vi "Write Tree Control Ref.vi"(8 "error in (no error)":errorcluster, 10 "Tag Tree Reference":refnum<vi>, 11 "Tag Tree Helper In":refnum<class "Tag Tree Helper.lvclass">) -> (0 "error out":errorcluster, 3 "Tag Tree Helper Out":refnum<class "Tag Tree Helper.lvclass">)   [LabVIEW 2020, in "Process Generation.lvlib" / "Tag Tree Helper.lvclass"]
uses:
  Tag Tree Helper.lvclass
  Tag Tree Helper.lvclass/Tag Tree Helper.ctl
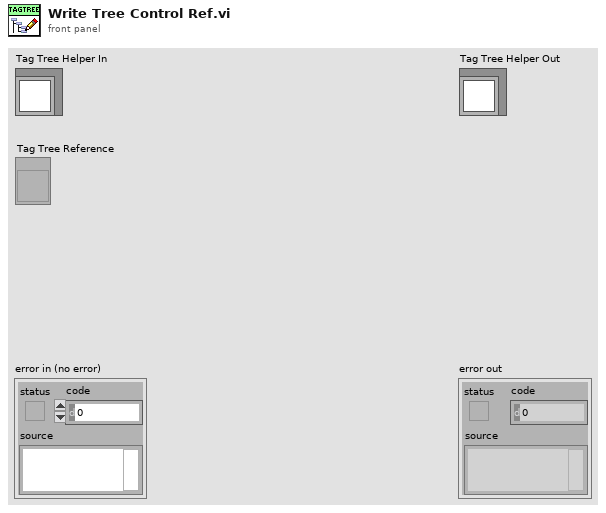
[diagram p1: front panel]
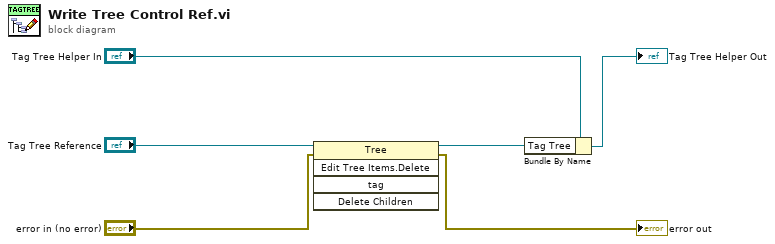
[diagram p0: block diagram]
diagram:
  n1 = invoke class="Tree" method="Edit Tree Items.Delete"(reference="Tag Tree Reference", error in="error in (no error)") -> (reference out=w3:refnum<vi>, error out=→"error out":errorcluster)  [unwired: 3 in, 3 out]
  n2 = Bundle By Name(cluster="Tag Tree Helper In", "Tag Tree"=w3) -> (→"Tag Tree Helper Out":refnum<class "Tag Tree Helper.lvclass">)
